vi "Add Message.vi"(0 "PainOutputTerminal in":refnum<class "PainOutputTerminal.lvclass">, 5 "Line Number":i64, 7 "Message":string, 11 "error in (no error)":errorcluster) -> (4 "PainOutputTerminal out":refnum<class "PainOutputTerminal.lvclass">, 15 "error out":errorcluster)   [LabVIEW 2016, in "PainOutputTerminal.lvclass"]
uses:
  PainOutputTerminal.lvclass
  PainOutputTerminal.lvclass/PainOutputTerminal.ctl
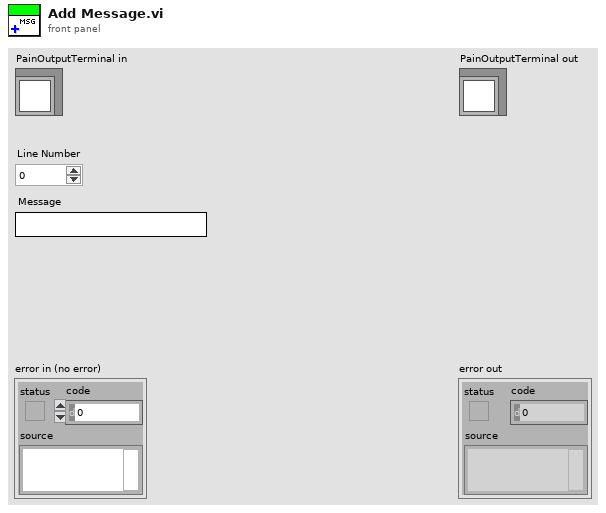
[diagram p1: front panel]
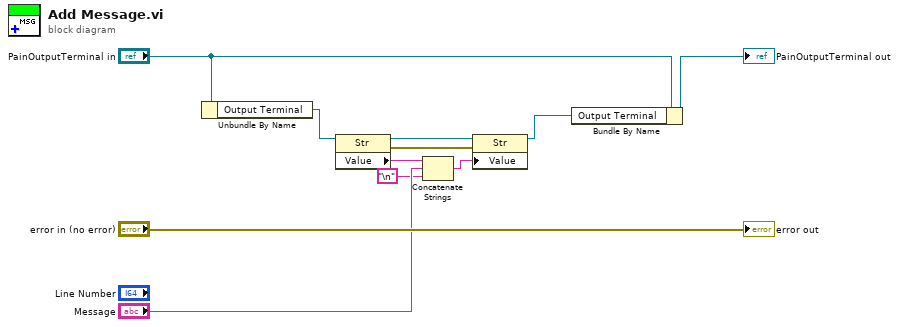
[diagram p0: block diagram]
diagram:
  n1 = Unbundle By Name("PainOutputTerminal in") -> ("Output Terminal"=w9:refnum<vi>)
  n2 = property class="Str"(reference=w9) -> (reference out=w8:refnum<vi>, error out=w10:errorcluster, "Value"=w6:string)  [unwired: 1 in]
  n3 = Concatenate Strings(w6, "Message", "\n" ("string")) -> (w5:string)
  n4 = property class="Str"(reference=w8, error in=w10, "Value"=w5) -> (reference out=w7:refnum<vi>)  [unwired: 1 out]
  n5 = Bundle By Name(cluster="PainOutputTerminal in", "Output Terminal"=w7) -> (→"PainOutputTerminal out":refnum<class "PainOutputTerminal.lvclass">)
  "error out" <- "error in (no error)"
